vi "信号持续时间参数配置.vi"(11 "标题":string) -> ()   [LabVIEW 2016, in "环境动力监测库.lvlib"]
panel:
  in  "信号持续时间":u32=60 format="%.0fS"
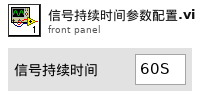
[diagram p1: front panel]
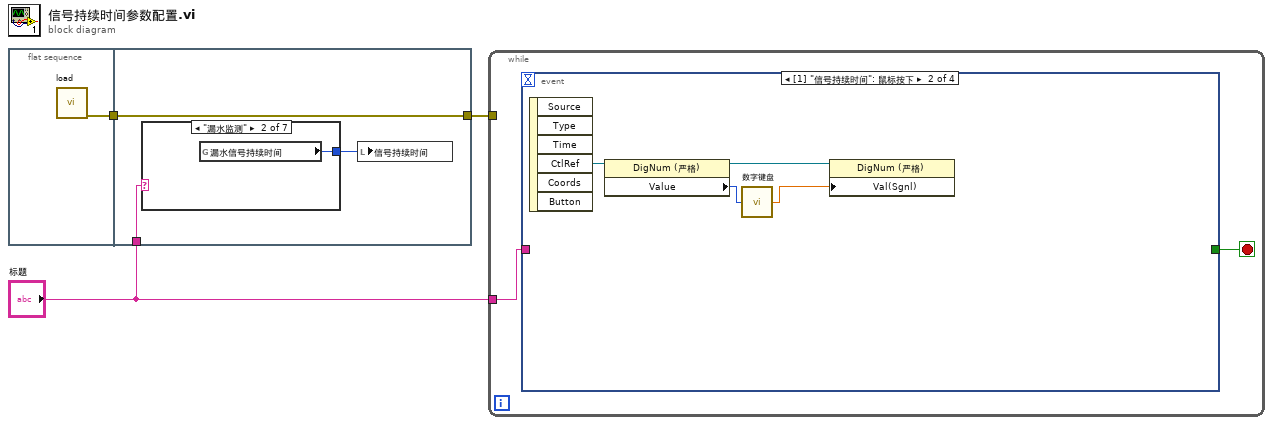
[diagram p0: block diagram]
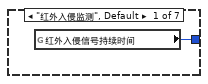
[diagram p2: hidden frame]
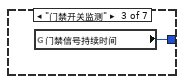
[diagram p3: hidden frame]
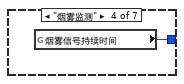
[diagram p4: hidden frame]
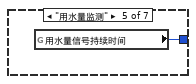
[diagram p5: hidden frame]
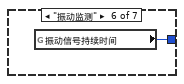
[diagram p6: hidden frame]
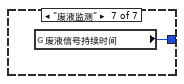
[diagram p7: hidden frame]
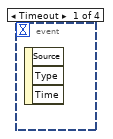
[diagram p8: hidden frame]
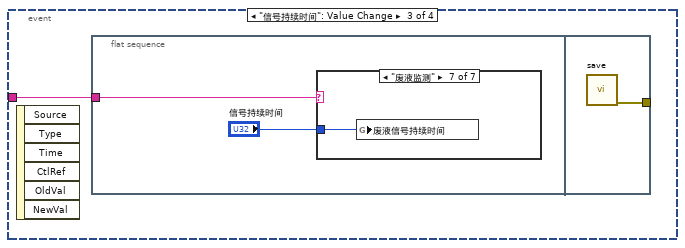
[diagram p9: hidden frame]
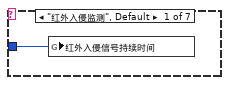
[diagram p10: hidden frame]
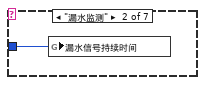
[diagram p11: hidden frame]
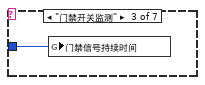
[diagram p12: hidden frame]
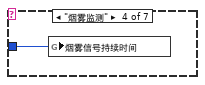
[diagram p13: hidden frame]
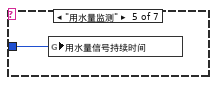
[diagram p14: hidden frame]
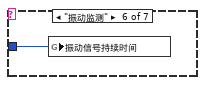
[diagram p15: hidden frame]
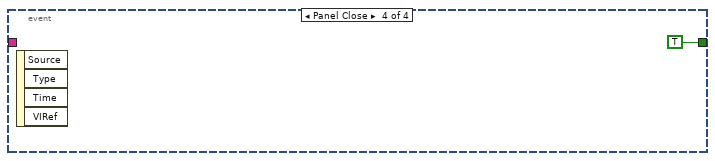
[diagram p16: hidden frame]
diagram:
  n1 = flat-sequence {
    tunnel: [w4] -> w3
    tunnel: [w7] -> w2
    tunnel: w3 -> [w7]
    tunnel: "标题" -> [w5]
    frame #0 {
      n2 = call "load.vi"() -> ("error out"=w4:errorcluster)  [unwired: 11 in]
    }
    frame #1 {
      n3 = case shown="\"漏水监测\"" w5 {
        tunnel: [w8 w9 w10 w11 w12 w13 w14] -> w6
        frame "红外入侵监测", Default {
          n4 = global read "断电保存全局变量.vi" "红外入侵信号持续时间"() -> (w8:u32)
        }
        frame "漏水监测" {
          n5 = global read "断电保存全局变量.vi" "漏水信号持续时间"() -> (w9:u32)
        }
        frame "门禁开关监测" {
          n6 = global read "断电保存全局变量.vi" "门禁信号持续时间"() -> (w10:u32)
        }
        frame "烟雾监测" {
          n7 = global read "断电保存全局变量.vi" "烟雾信号持续时间"() -> (w11:u32)
        }
        frame "用水量监测" {
          n8 = global read "断电保存全局变量.vi" "用水量信号持续时间"() -> (w12:u32)
        }
        frame "振动监测" {
          n9 = global read "断电保存全局变量.vi" "振动信号持续时间"() -> (w13:u32)
        }
        frame "废液监测" {
          n10 = global read "断电保存全局变量.vi" "废液信号持续时间"() -> (w14:u32)
        }
      }
      n11 = local write "信号持续时间"(w6) -> ()
    }
  }
  n12 = while {
    tunnel: w2 -> [_]
    tunnel: "标题" -> [w15]
    stop <- w16 stop-if-true
    n13 = event shown="[1] \"信号持续时间\": 鼠标按下" {
      selector: _ -> [_ _ _ _]
      dyn-events: _ -> [_ _ _ _]
      timeout: _ -> [_ _ _ _]
      tunnel: [_ _ _ TRUE] -> w16
      tunnel: w15 -> [_ _ w21 _]
      event Timeout {
        n14 = event-data() -> ()  [unwired: 1 in, 3 out]
      }
      event "信号持续时间": Mouse Down {
        n15 = event-data() -> ("CtlRef"=w17:refnum<vi>)  [unwired: 1 in, 5 out]
        n16 = property class="DigNum (严格)"(reference=w17) -> (reference out=w19:refnum<vi>, "Value"=w20:u32)  [unwired: 1 in, 1 out]
        n17 = call "数字键盘.vi"("OldNumber"=w20) -> ("NewNumber"=w18:sgl)
        n18 = property class="DigNum (严格)"(reference=w19, "Val(Sgnl)"=w18) -> ()  [unwired: 1 in, 2 out]
      }
      event "信号持续时间": Value Change {
        n19 = event-data() -> ()  [unwired: 1 in, 6 out]
        n20 = flat-sequence {
          tunnel: w21 -> [w23]
          tunnel: [w31] -> _
          frame #0 {
            n21 = case shown="\"废液监测\"" w23 {
              tunnel: "信号持续时间" -> [w24 w25 w26 w27 w28 w29 w30]
              frame "红外入侵监测", Default {
                n22 = global write "断电保存全局变量.vi" "红外入侵信号持续时间"(w24) -> ()
              }
              frame "漏水监测" {
                n23 = global write "断电保存全局变量.vi" "漏水信号持续时间"(w25) -> ()
              }
              frame "门禁开关监测" {
                n24 = global write "断电保存全局变量.vi" "门禁信号持续时间"(w26) -> ()
              }
              frame "烟雾监测" {
                n25 = global write "断电保存全局变量.vi" "烟雾信号持续时间"(w27) -> ()
              }
              frame "用水量监测" {
                n26 = global write "断电保存全局变量.vi" "用水量信号持续时间"(w28) -> ()
              }
              frame "振动监测" {
                n27 = global write "断电保存全局变量.vi" "振动信号持续时间"(w29) -> ()
              }
              frame "废液监测" {
                n28 = global write "断电保存全局变量.vi" "废液信号持续时间"(w30) -> ()
              }
            }
          }
          frame #1 {
            n29 = call "save.vi"() -> ("error out"=w31:errorcluster)  [unwired: 11 in]
          }
        }
      }
      event Panel Close {
        n30 = event-data() -> ()  [unwired: 1 in, 4 out]
      }
    }
  }
